vi "Read Setpoint.vi"   [LabVIEW 2022 SP3, in "Bronkhorst FLOW-BUS.lvlib"]
doc: "Reads the setpoint value in the instrument. The setpoint is used to tell the PID controller in the instrument what the wanted amount of mass flow or pressure is."
uses:
  Bronkhorst FLOW-BUS.lvlib
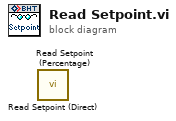
[diagram p0: block diagram]
diagram:
  n1 = call "Read Setpoint (Direct).vi"() -> ()  [unwired: 9 in, 3 out]
  n2 = call "Read Setpoint (Percentage).vi"() -> ()  [unwired: 9 in, 3 out]
